vi "Sub_Preprocessing_FEA_Frequency_Bounds.vi"(2 "FEA Parameters":T1={"LEMP"={"Eigenvalues"=[], "Square Transpose Eigenvectors"=[], "1/deltaStiff"=0.0}, "nodes of interest"=[], "all nodes"=[], "Eigenvalue Method"=enum."0-Local Eigen Modification Procedure", "Mode Count"=3, "initial_pin_node"=0, "Sub Sample"=TRUE}, 3 "Modeling Parameters":T2) -> (0 "FEA Parameters":T1, 1 "Modeling Parameters":T2)   [LabVIEW 2021]
panel:
  out "Waveform Graph":dynamicdata(graph)
  out "third modes":dbl[](array[numeric])
  out "first modes":dbl[](array[numeric])
  out "second modes":dbl[](array[numeric])
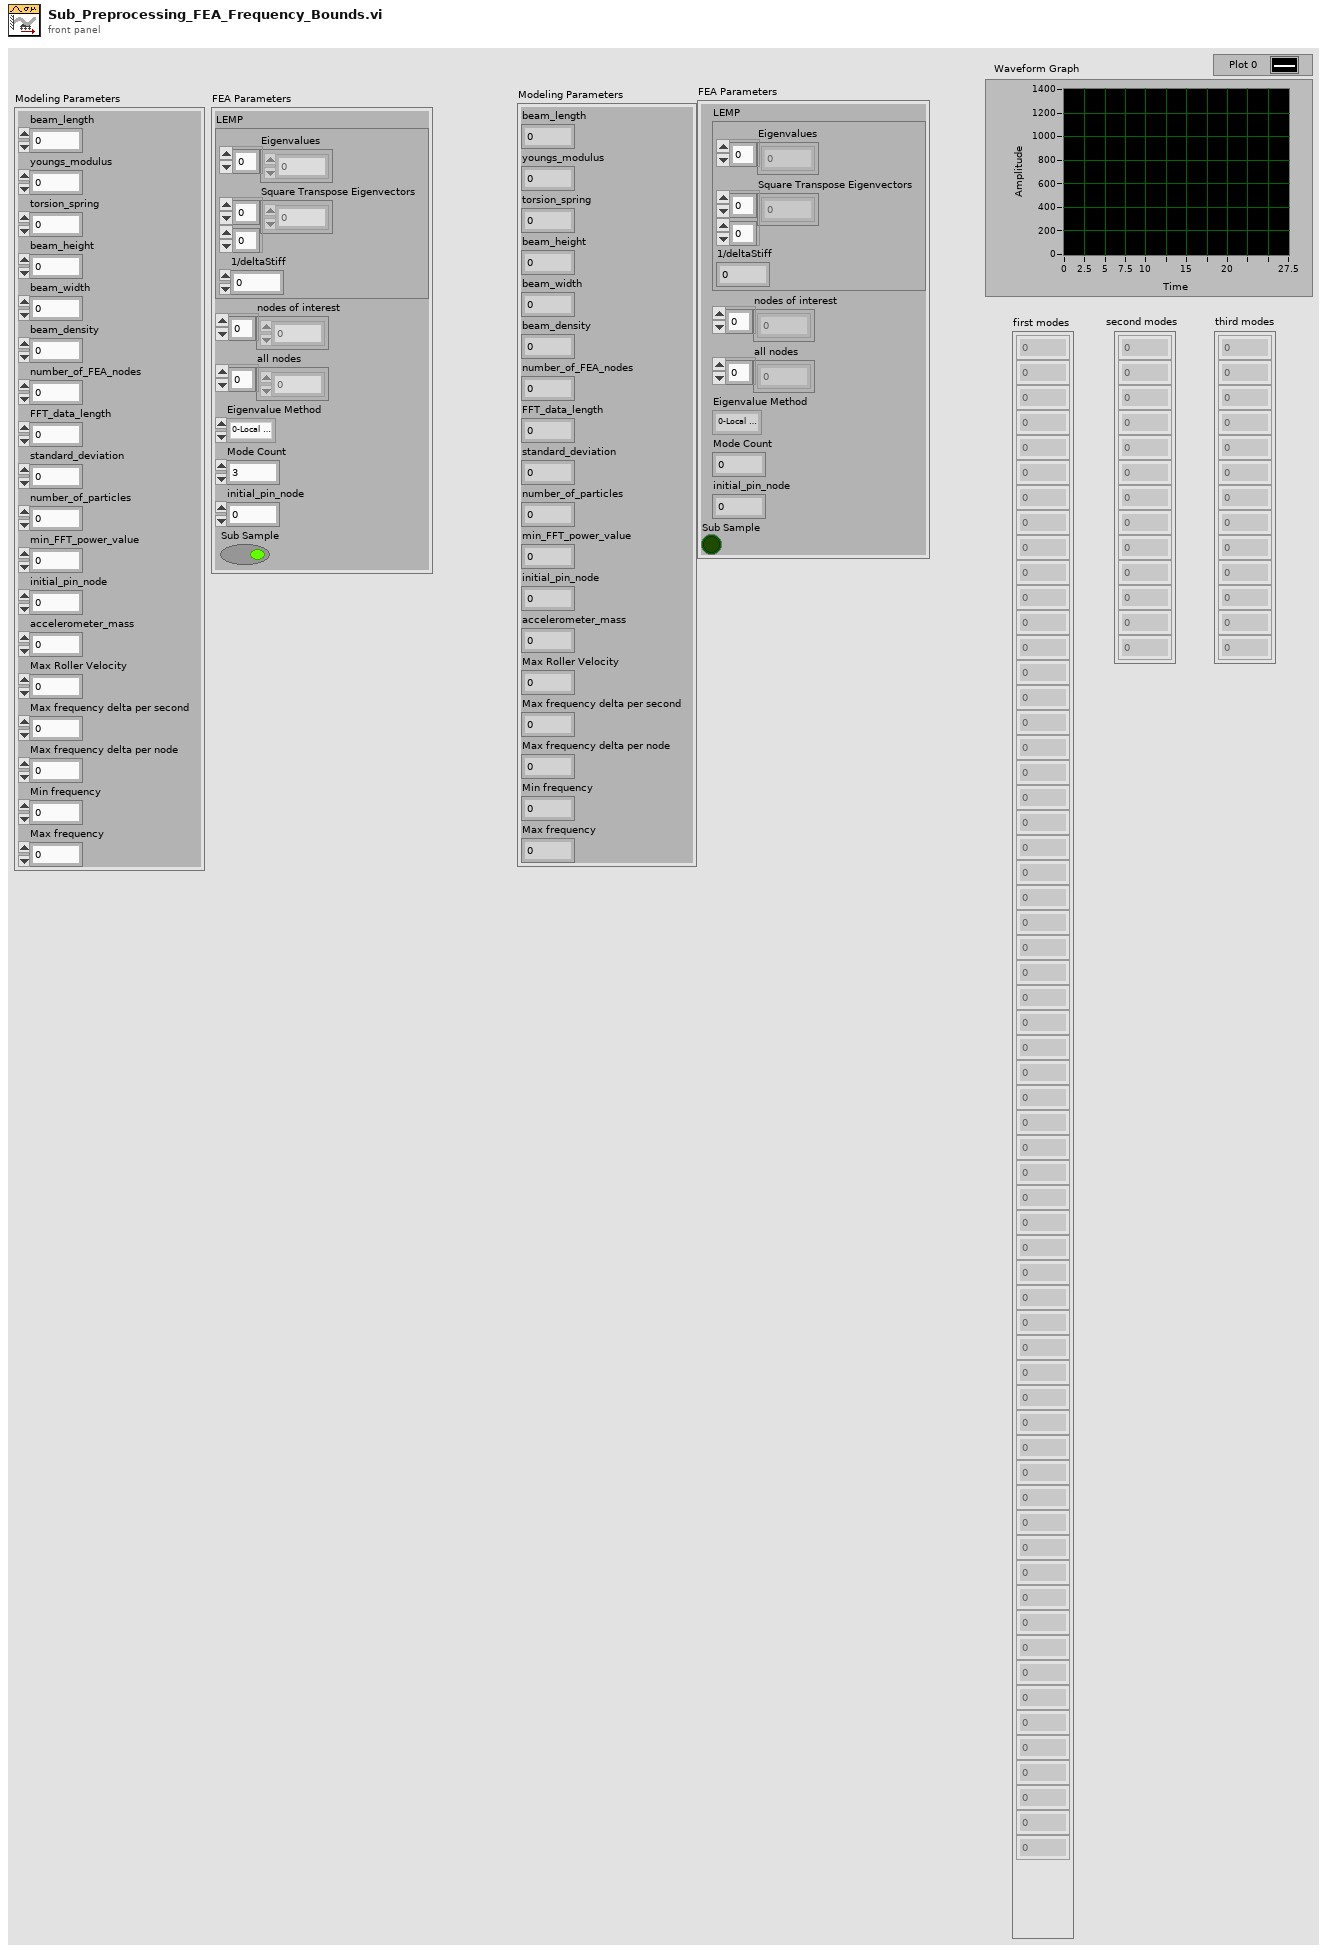
[diagram p1: front panel]
types:
  T1 = cluster{"LEMP":cluster{"Eigenvalues":dbl[], "Square Transpose Eigenvectors":dbl[][], "1/deltaStiff":dbl}, "nodes of interest":i32[], "all nodes":i32[], "Eigenvalue Method":enum16{"0-Local Eigen Modification Procedure", "1-LabVIEW generalized eigenvalues", "2-LabVIEW M^-1K eigenvalues", "3-LabVIEW Cholesky Factorization", "4-Cholesky Factorization CPU SGL", "5-Cholesky Factorization CPU FXP", "6-Cholesky Factorization FPGA SGL", "7-Cholesky Factorization FPGA SGL SCL"}, "Mode Count":i32, "initial_pin_node":i32, "Sub Sample":bool}
  T2 = cluster{"beam_length":dbl, "youngs_modulus":dbl, "torsion_spring":dbl, "beam_height":dbl, "beam_width":dbl, "beam_density":dbl, "number_of_FEA_nodes":i32, "FFT_data_length":i32, "standard_deviation":dbl, "number_of_particles":i32, "min_FFT_power_value":dbl, "initial_pin_node":i32, "accelerometer_mass":dbl, "Max Roller Velocity":dbl, "Max frequency delta per second":dbl, "Max frequency delta per node":dbl, "Min frequency":dbl, "Max frequency":dbl}
  T3 = cluster{"Eigenvalues":dbl[], "Square Transpose Eigenvectors":dbl[][], "1/deltaStiff":dbl}
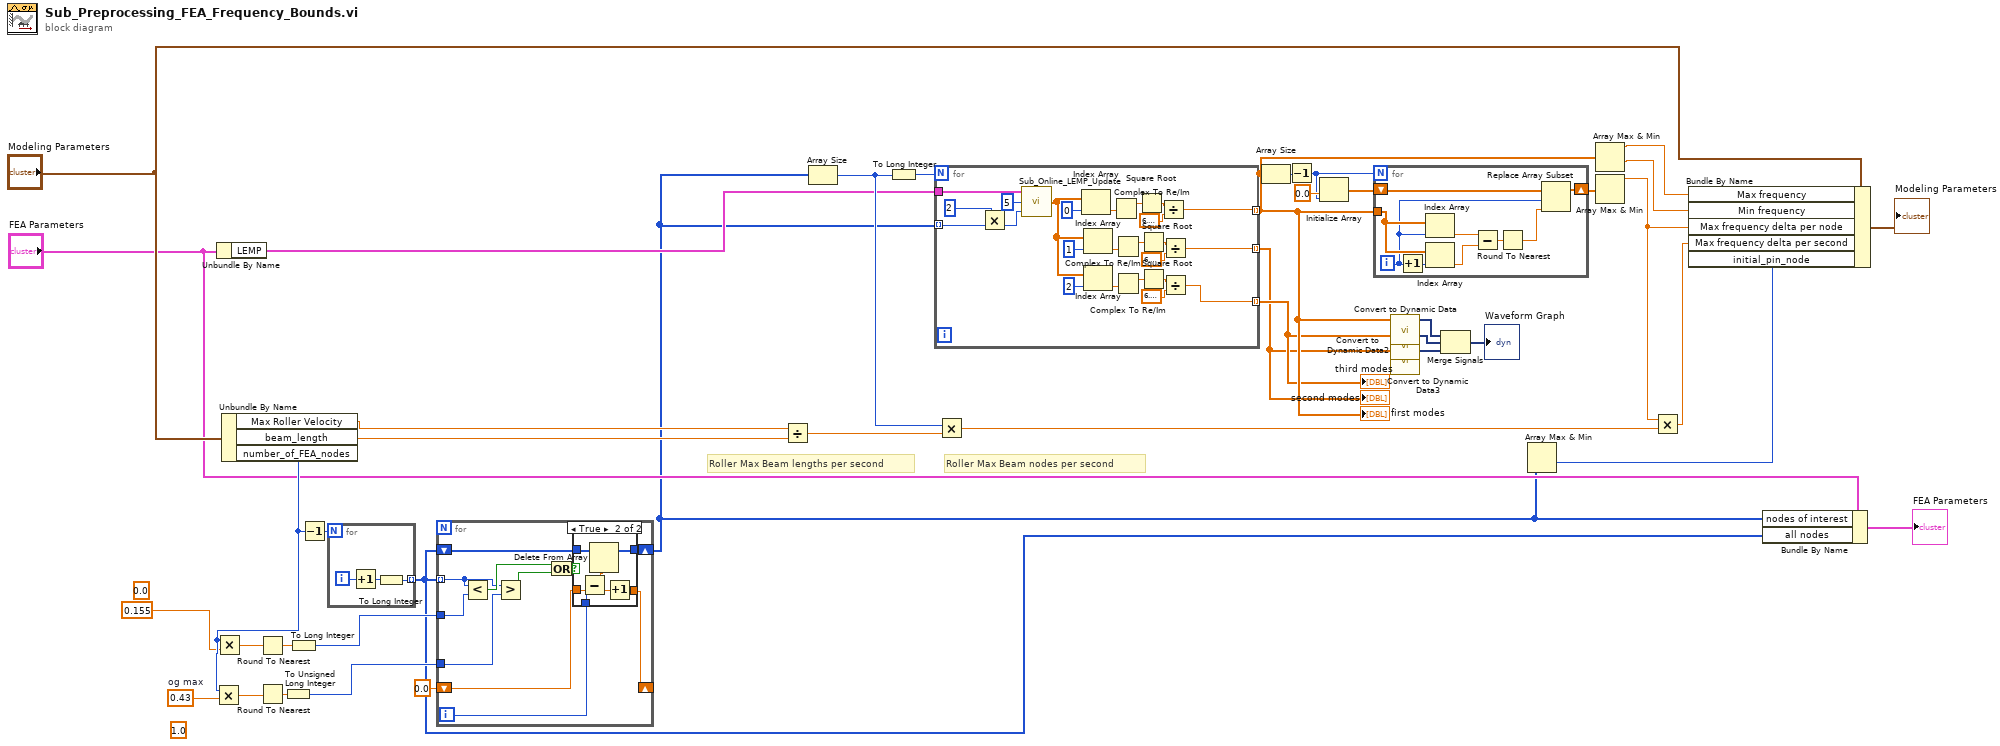
[diagram p0: block diagram]
diagram:
  (unwired) 0.0
  (unwired) 1.0
  w3 = 0.43  # og max
  # "Roller Max Beam nodes per second"
  # "Roller Max Beam lengths per second"
  n1 = Unbundle By Name("FEA Parameters") -> ("LEMP"=w16:T3)
  n2 = Unbundle By Name("Modeling Parameters") -> ("Max Roller Velocity"=w39:dbl, "beam_length"=w38:dbl, "number_of_FEA_nodes"=w32:i32)
  n3 = Multiply(x=w32, y=w3) -> (x*y=w31:dbl)
  n4 = Multiply(x=w32, y=0.155) -> (x*y=w30:dbl)
  n5 = Round To Nearest(number=w30) -> (nearest integer value=w29:dbl)
  n6 = Round To Nearest(number=w31) -> (nearest integer value=w28:dbl)
  n7 = To Unsigned Long Integer(number=w28) -> (unsigned 32bit integer=w27:u32)
  n8 = To Long Integer(number=w29) -> (32bit integer=w26:i32)
  n9 = Decrement(x=w32) -> (x-1=w35:i32)
  n10 = for {
    N: w35 -> [_]
    tunnel: [w44] -> w23 mode=indexing
    i -> [w42]
    n11 = Increment(x=w42) -> (x+1=w43:i32)
    n12 = To Long Integer(number=w43) -> (32bit integer=w44:i32)
  }
  n13 = for {
    tunnel: w23 -> [w48] mode=indexing
    shift-right: [w51] -> w2
    shift-left: w23 -> [w55]
    shift-right: [w50] -> _
    shift-left: 0.0 -> [w49]
    tunnel: w26 -> [w46]
    tunnel: w27 -> [w45]
    i -> [w47]
    n14 = Less?(x=w48, y=w46) -> (x < y?=w52:bool)
    n15 = Greater?(x=w48, y=w45) -> (0:w54:bool)
    n16 = Or(x=w52, y=w54) -> (x .or. y?=w53:bool)
    n17 = case shown="True" w53 {
      tunnel: w55 -> [w57 w62]
      tunnel: [w57 w63] -> w51
      tunnel: [w56 w61] -> w50
      tunnel: w49 -> [w56 w60]
      tunnel: w47 -> [_ w59]
      frame False {
      }
      frame True {
        n18 = Subtract(x=w59, y=w60) -> (x-y=w58:dbl)
        n19 = Delete From Array(array=w62, index=w58) -> (array with subset deleted=w63:i32[])  [unwired: 1 in, 1 out]
        n20 = Increment(x=w60) -> (x+1=w61:dbl)
      }
    }
  }
  n21 = Divide(x=w39, y=w38) -> (x/y=w41:dbl)
  n22 = Array Size(array=w2) -> (size(s)=w33:i32)
  n23 = To Long Integer(number=w33) -> (32bit integer=w5:i32)
  n24 = for {
    N: w5 -> [_]
    tunnel: w16 -> [w85]
    tunnel: [w78] -> w9 mode=indexing
    tunnel: [w72] -> w7 mode=indexing
    tunnel: [w65] -> w8 mode=indexing
    tunnel: w2 -> [w64] mode=indexing
    n25 = Multiply(x=2, y=w64) -> (x*y=w84:i32)
    n26 = call "Sub_Online_LEMP_Update.vi"("Effected DOF"=w84, "Mode count"=5, "LEMP"=w85) -> ("Updated Eigenvalues"=w66:dbl[])
    n27 = Index Array(array=w66, index=0) -> (element=w82:dbl)
    n28 = Index Array(array=w66, index=1) -> (element=w77:dbl)
    n29 = Index Array(array=w66, index=2) -> (element=w71:dbl)
    n30 = Complex To Re/Im(x + iy=w82) -> (x=w81:dbl)  [unwired: 1 out]
    n31 = Complex To Re/Im(x + iy=w77) -> (x=w76:dbl)  [unwired: 1 out]
    n32 = Complex To Re/Im(x + iy=w71) -> (x=w70:dbl)  [unwired: 1 out]
    n33 = Square Root(x=w81) -> (sqrt(x)=w80:dbl)
    n34 = Square Root(x=w76) -> (sqrt(x)=w75:dbl)
    n35 = Square Root(x=w70) -> (sqrt(x)=w69:dbl)
    n36 = Divide(x=w80, y=6.283185307179586) -> (x/y=w78:dbl)
    n37 = Divide(x=w75, y=6.283185307179586) -> (x/y=w72:dbl)
    n38 = Divide(x=w69, y=6.283185307179586) -> (x/y=w65:dbl)
  }
  "second modes" <- w7
  "first modes" <- w9
  "third modes" <- w8
  n39 = Multiply(x=w33, y=w41) -> (x*y=w40:dbl)
  n40 = Array Size(array=w9) -> (size(s)=w21:i32)
  n41 = Decrement(x=w21) -> (x-1=w18:i32)
  n42 = Initialize Array(0.0 ("element"), w18) -> (w20:dbl[])
  n43 = for {
    N: w18 -> [_]
    tunnel: w9 -> [w96]
    shift-right: [w90] -> w17
    shift-left: w20 -> [w91]
    i -> [w89]
    n44 = Increment(x=w89) -> (x+1=w95:i32)
    n45 = Index Array(array=w96, index=w89) -> (element=w94:dbl)
    n46 = Index Array(array=w96, index=w95) -> (element=w93:dbl)
    n47 = Subtract(x=w94, y=w93) -> (x-y=w92:dbl)
    n48 = Round To Nearest(number=w92) -> (nearest integer value=w88:dbl)
    n49 = Replace Array Subset(array=w91, new element=w88, index=w89) -> (w90:dbl[])
  }
  n50 = call "Convert to Dynamic Data"("Array"=w9) -> ("Dynamic Data Type"=w12:dynamicdata)  [unwired: 3 in]
  n51 = call "Convert to Dynamic Data2"("Array"=w8) -> ("Dynamic Data Type"=w11:dynamicdata)  [unwired: 3 in]
  n52 = call "Convert to Dynamic Data3"("Array"=w7) -> ("Dynamic Data Type"=w10:dynamicdata)  [unwired: 3 in]
  n53 = Merge Signals(w12, w11, w10) -> (→"Waveform Graph":dynamicdata)
  n54 = Array Max & Min(array=w2) -> (min value=w1:i32)  [unwired: 3 out]
  n55 = Array Max & Min(array=w9) -> (max value=w15:dbl, min value=w14:dbl)  [unwired: 2 out]
  n56 = Array Max & Min(array=w17) -> (max value=w13:dbl)  [unwired: 3 out]
  n57 = Multiply(x=w13, y=w40) -> (x*y=w36:dbl)
  n58 = Bundle By Name(cluster="Modeling Parameters", "Max frequency"=w15, "Min frequency"=w14, "Max frequency delta per node"=w13, "Max frequency delta per second"=w36, "initial_pin_node"=w1) -> (→"Modeling Parameters":T2)
  n59 = Bundle By Name(cluster="FEA Parameters", "nodes of interest"=w2, "all nodes"=w23) -> (→"FEA Parameters":T1)
